vi "cstring_free_memory.vi"(8 "error in (no error)":errorcluster, 11 "ptr":u64) -> (0 "error out":errorcluster)   [LabVIEW 2021, in "TOML2JSON.lvlib"]
uses:
  TOML2JSON.lvlib
  include/TOML2JSON_64.dll
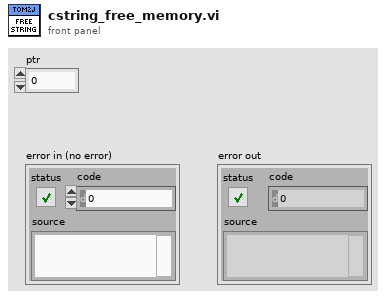
[diagram p1: front panel]
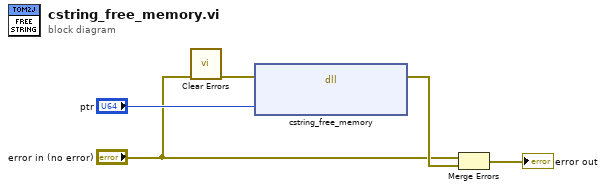
[diagram p0: block diagram]
diagram:
  n1 = call <vilib>:"Clear Errors.vi"("error in (no error)"="error in (no error)") -> ("error out"=w4:errorcluster)  [unwired: 5 in, 1 out]
  n2 = dll-call lib="C:/GIT checkouts/LabVIEW-Kraken/Framework_Code/VIPs/TOML2JSON/lv_src/include/TOML2JSON_*.dll" fn="cstring_free_memory"(error in=w4, "ptr"="ptr") -> (error out=w3:errorcluster)  [unwired: 4 in, 1 out]
  n3 = Merge Errors("error in (no error)", w3) -> (→"error out":errorcluster)
